vi "Create Channel Array.vi"(8 "error in":errorcluster, 10 "channel settings":T1[](array[typedef]), 11 "counter input pwm mode in":refnum<class "Counter Input PWM Mode.lvclass">) -> (0 "error out":errorcluster, 2 "channels":refnum<class "PWM Input Channel.lvclass">[](array[class]), 3 "counter input pwm mode out":refnum<class "Counter Input PWM Mode.lvclass">)   [LabVIEW 2017, in "Scan Engine Scripting.lvlib" / "Counter Input PWM Mode.lvclass"]
uses:
  Counter Input PWM Mode.lvclass
  Channel Classes/PWM Input Channel/PWM Input Channel.lvclass
  Controls/counter input pwm channel settings.ctl
  Channel Classes/PWM Input Channel/Measurement Type.ctl
  Scan Engine Scripting.lvlib
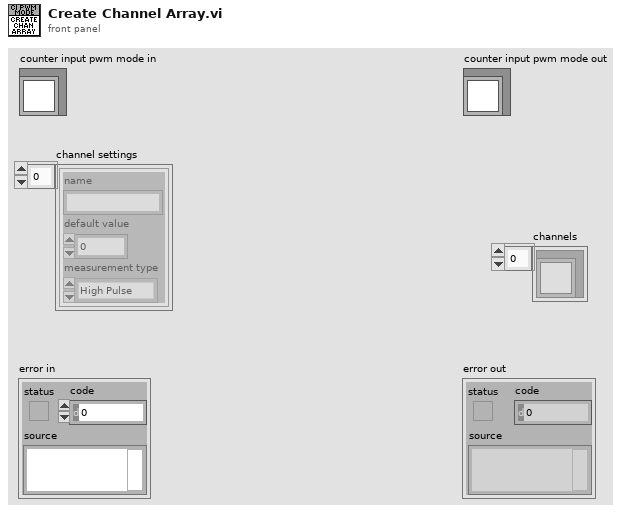
[diagram p1: front panel]
types:
  T1 = typedef "Scan Engine Scripting.lvlib/counter input pwm channel settings.ctl" = cluster{"name":string, "default value":dbl, "measurement type":T2}
  T2 = typedef "Scan Engine Scripting.lvlib/PWM Input Channel.lvclass/Measurement Type.ctl" = enum16{"High Pulse", "Low Pulse", "Most Recent"}
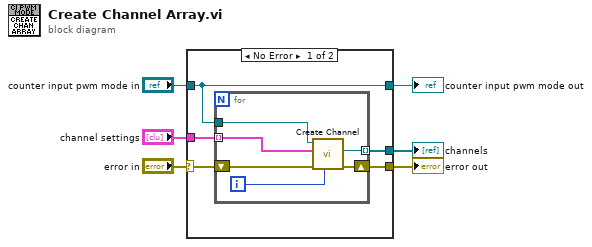
[diagram p0: block diagram]
diagram:
  n1 = case shown="No Error" "error in" {
    selector: "error in" -> [w10 w19]
    tunnel: [w9 w19] -> w4
    tunnel: [w11 w18] -> w1
    tunnel: "counter input pwm mode in" -> [w11 w18]
    tunnel: "channel settings" -> [w8 _]
    tunnel: [w7 _] -> w6
    frame No Error {
      n2 = for {
        tunnel: w11 -> [w17]
        tunnel: w8 -> [w12] mode=indexing
        shift-right: [w15] -> w9
        shift-left: w10 -> [w16]
        tunnel: [w13] -> w7 mode=indexing
        i -> [w14]
        n3 = call "Create Channel.vi"("index"=w14, "error in"=w16, "channel settings"=w12, "counter input pwm mode in"=w17) -> ("error out"=w15:errorcluster, "channel out"=w13:refnum<class "PWM Input Channel.lvclass">)  [unwired: 5 in, 1 out]
      }
    }
    frame Error {
    }
  }
  "error out" <- w4
  "counter input pwm mode out" <- w1
  "channels" <- w6
